vi "find pre-exec timing tag indices.vi"(8 "error in":errorcluster, 10 "execution timing tags":T2, 11 "data dictionary in":refnum<class "data dictionary.lvclass">) -> (0 "error out":errorcluster, 3 "exec timing indices":T1)   [LabVIEW 2013, in "Standard Engine Runtime.lvclass"]
doc: "Locates tags, if specified, for timing information. If the tags aren't found, -1 is used and that tag is disabled."
uses:
  Standard Engine Runtime.lvclass
  <vilib>/NI/Tag Bus/dictionary/data dictionary.lvclass
  Configuration/execution timing tags.ctl
  main engine/execution timing indices.ctl
  <vilib>/NI/Tag Bus/dictionary/data dictionary.lvclass/data dictionary.ctl
  <vilib>/NI/Tag Bus/dictionary/lookup polymorphs/locate double.vi
  <vilib>/NI/Tag Bus/dictionary/search/find data index.vi
  <vilib>/NI/Tag Bus/dictionary/search/search string list.vi
  <vilib>/NI/Tag Bus/dictionary/tag not found.vi
  main engine/main engine.lvlib
  Configuration/Standard Engine Configuration.lvclass
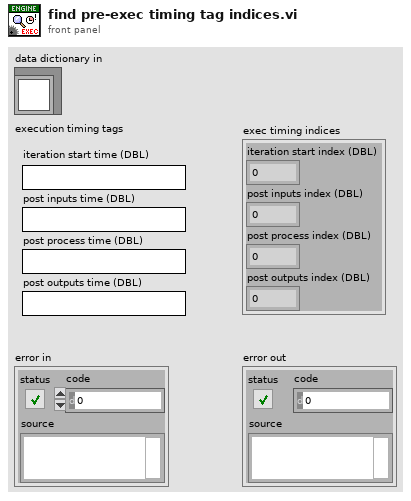
[diagram p1: front panel]
types:
  T1 = typedef "main engine.lvlib/execution timing indices.ctl" = cluster{"iteration start index (DBL)":i32, "post inputs index (DBL)":i32, "post process index (DBL)":i32, "post outputs index (DBL)":i32}
  T2 = typedef "Standard Engine Configuration.lvclass/execution timing tags.ctl" = cluster{"iteration start time (DBL)":string, "post inputs time (DBL)":string, "post process time (DBL)":string, "post outputs time (DBL)":string}
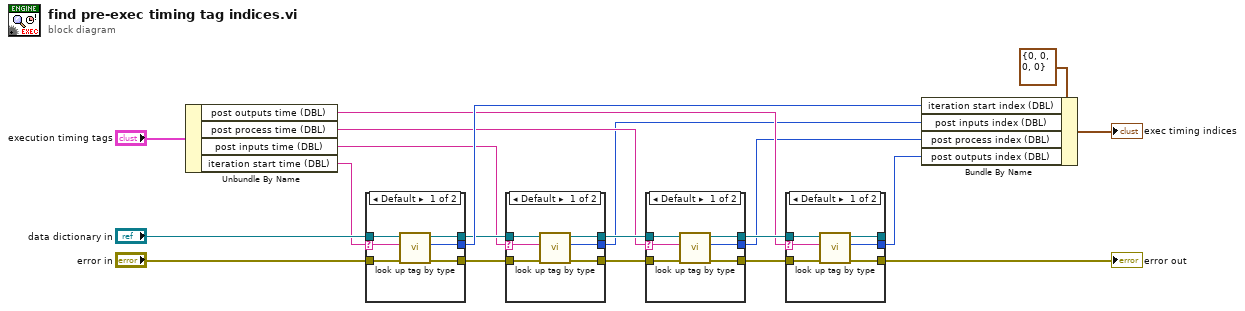
[diagram p0: block diagram]
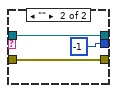
[diagram p2: hidden frame]
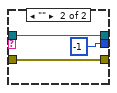
[diagram p3: hidden frame]
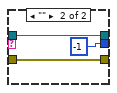
[diagram p4: hidden frame]
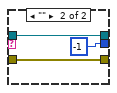
[diagram p5: hidden frame]
diagram:
  n1 = Unbundle By Name("execution timing tags") -> ("post outputs time (DBL)"=w5:string, "post process time (DBL)"=w6:string, "post inputs time (DBL)"=w7:string, "iteration start time (DBL)"=w17:string)
  n2 = case shown="Default" w17 {
    selector: w17 -> [w22 _]
    tunnel: [w25 w29] -> w12
    tunnel: "error in" -> [w26 w29]
    tunnel: "data dictionary in" -> [w23 w28]
    tunnel: [w24 w28] -> w13
    tunnel: [w21 -1] -> w14
    frame Default {
      n3 = call-poly <vilib>:"look up tag by type.vi"("error in"=w26, "name"=w22, "data dictionary in"=w23) -> ("error out"=w25:errorcluster, "index"=w21:i32, "data dictionary out"=w24:refnum<class "data dictionary.lvclass">)  [unwired: 6 in]
    }
    frame "" {
    }
  }
  n4 = case shown="Default" w7 {
    selector: w7 -> [w31 _]
    tunnel: [w34 w38] -> w11
    tunnel: w12 -> [w35 w38]
    tunnel: w13 -> [w32 w37]
    tunnel: [w33 w37] -> w9
    tunnel: [w30 -1] -> w4
    frame Default {
      n5 = call-poly <vilib>:"look up tag by type.vi"("error in"=w35, "name"=w31, "data dictionary in"=w32) -> ("error out"=w34:errorcluster, "index"=w30:i32, "data dictionary out"=w33:refnum<class "data dictionary.lvclass">)  [unwired: 6 in]
    }
    frame "" {
    }
  }
  n6 = case shown="Default" w6 {
    selector: w6 -> [w40 _]
    tunnel: [w43 w47] -> w10
    tunnel: w11 -> [w44 w47]
    tunnel: w9 -> [w41 w46]
    tunnel: [w42 w46] -> w8
    tunnel: [w39 -1] -> w3
    frame Default {
      n7 = call-poly <vilib>:"look up tag by type.vi"("error in"=w44, "name"=w40, "data dictionary in"=w41) -> ("error out"=w43:errorcluster, "index"=w39:i32, "data dictionary out"=w42:refnum<class "data dictionary.lvclass">)  [unwired: 6 in]
    }
    frame "" {
    }
  }
  n8 = case shown="Default" w5 {
    selector: w5 -> [w49 _]
    tunnel: [w52 w56] -> w1
    tunnel: w10 -> [w53 w56]
    tunnel: w8 -> [w50 w55]
    tunnel: [w51 w55] -> _
    tunnel: [w48 -1] -> w2
    frame Default {
      n9 = call-poly <vilib>:"look up tag by type.vi"("error in"=w53, "name"=w49, "data dictionary in"=w50) -> ("error out"=w52:errorcluster, "index"=w48:i32, "data dictionary out"=w51:refnum<class "data dictionary.lvclass">)  [unwired: 6 in]
    }
    frame "" {
    }
  }
  "error out" <- w1
  n10 = Bundle By Name(cluster=T1 {"iteration start index (DBL)"=0, "post inputs index (DBL)"=0, "post process index (DBL)"=0, "post outputs index (DBL)"=0} ("pre-execution timing"), "iteration start index (DBL)"=w14, "post inputs index (DBL)"=w4, "post process index (DBL)"=w3, "post outputs index (DBL)"=w2) -> (→"exec timing indices":T1)
